vi "_Veritech_LVCM_RunInterface.vi"(8 "error in (no error)":errorcluster) -> (0 "error out":errorcluster)   [LabVIEW 2014]
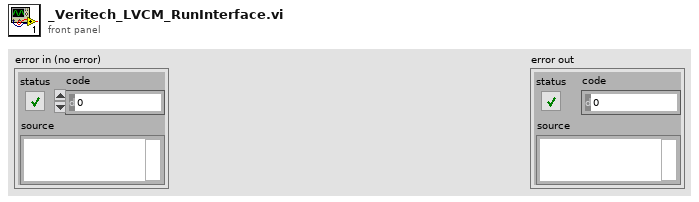
[diagram p1: front panel]
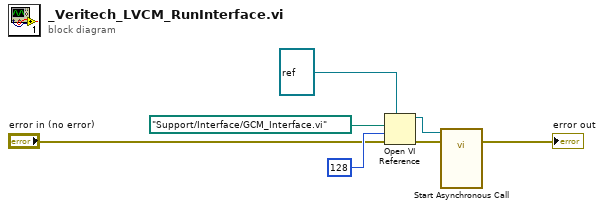
[diagram p0: block diagram]
diagram:
  n1 = Open VI Reference(type specifier VI Refnum (for type only)=refnum<vi> refnum, vi path=path "Support/Interface/GCM_Interface.vi", options=128, error in (no error)="error in (no error)") -> (vi reference=w6:refnum<vi>, error out=w7:errorcluster)  [unwired: 2 in]
  n2 = call-by-ref "Start Asynchronous Call"(reference=w6, error in=w7) -> (error out=→"error out":errorcluster)  [unwired: 12 in, 1 out]
